vi "LabVIEW example.vi"() -> ()   [LabVIEW 2025]
panel:
  out "distance":dbl
  in  "path to image file":path
  out "Intensity Graph":u8[][](graph)
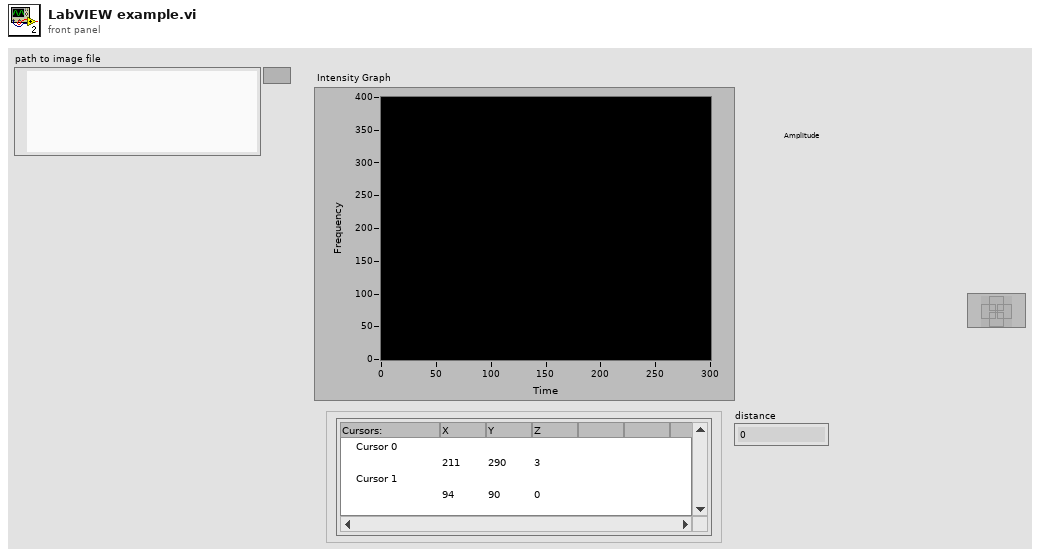
[diagram p1: front panel]
types:
  T1 = typedef "imagedata.ctl" = cluster{"image type":i32, "image depth":i32, "image":u8[], "mask":u8[], "colors":u32[], "Rectangle":cluster{"left":i16, "top":i16, "right":i16, "bottom":i16}}
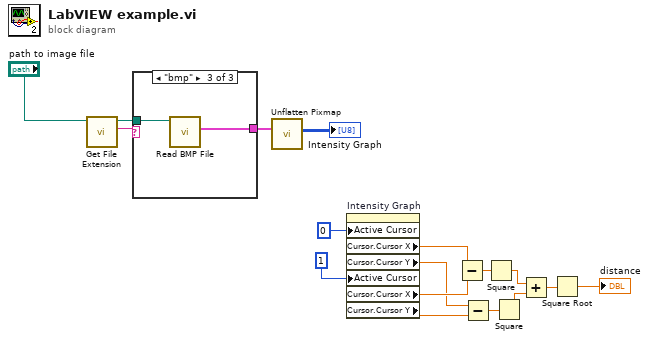
[diagram p0: block diagram]
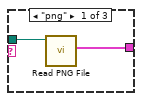
[diagram p2: hidden frame]
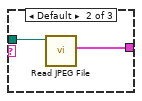
[diagram p3: hidden frame]
diagram:
  n1 = call <vilib>:"Get File Extension.vi"("file"="path to image file") -> ("lowercase file extension"=w15:string, "dup file"=w16:path)  [unwired: 6 in, 3 out]
  n2 = case shown="\"bmp\"" w15 {
    tunnel: w16 -> [w19 w21 w23]
    tunnel: [w18 w20 w22] -> w14
    frame "png" {
      n3 = call <vilib>:"Read PNG File.vi"("path to PNG file"=w19) -> ("image data"=w18:T1)  [unwired: 8 in, 2 out]
    }
    frame Default {
      n4 = call <vilib>:"Read JPEG File.vi"("path to JPEG file"=w21) -> ("image data"=w20:T1)  [unwired: 8 in, 2 out]
    }
    frame "bmp" {
      n5 = call <vilib>:"Read BMP File.vi"("path to BMP file"=w23) -> ("image data"=w22:T1)  [unwired: 8 in, 2 out]
    }
  }
  n6 = call <vilib>:"Unflatten Pixmap.vi"("image data"=w14) -> ("8-bit pixmap"=→"Intensity Graph":u8[][])  [unwired: 4 in, 6 out]
  n7 = property on="Intensity Graph" class="IntGraph (strict)"("Active Cursor"=u32 0, "Active Cursor"=u32 1) -> ("Cursor.Cursor X"=w10:dbl, "Cursor.Cursor Y"=w8:dbl, "Cursor.Cursor X"=w9:dbl, "Cursor.Cursor Y"=w7:dbl)  [unwired: 2 in, 2 out]
  n8 = Subtract(x=w10, y=w9) -> (x-y=w6:dbl)
  n9 = Subtract(x=w8, y=w7) -> (x-y=w5:dbl)
  n10 = Square(x=w6) -> (x^2=w3:dbl)
  n11 = Square(x=w5) -> (x^2=w4:dbl)
  n12 = Add(x=w3, y=w4) -> (x+y=w2:dbl)
  n13 = Square Root(x=w2) -> (sqrt(x)=→"distance":dbl)
